vi "Get Visibility.vi"(8 "error in (no error)":errorcluster, 11 "Panel in":refnum<class "Panel.lvclass">) -> (0 "error out":errorcluster, 2 "Visible":bool, 3 "Panel out":refnum<class "Panel.lvclass">)   [LabVIEW 2018]
uses:
  Panel.lvclass
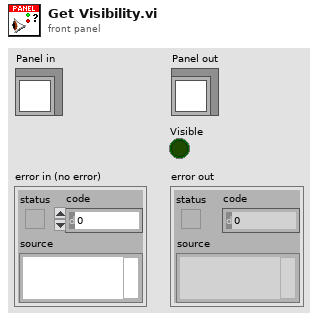
[diagram p1: front panel]
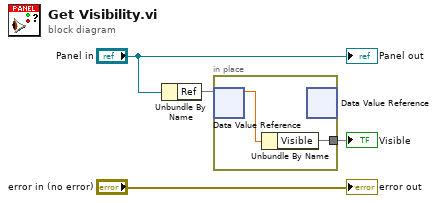
[diagram p0: block diagram]
diagram:
  n1 = Unbundle By Name("Panel in") -> ("Ref"=w3)
  n2 = in-place {
    in-place-border: [w5] -> w1
    n3 = in-place-dvr #1(w3) -> (w6:dbl)  [unwired: 1 out]
    n4 = Unbundle By Name(w6) -> ("Visible"=w5)
    n5 = in-place-dvr #1() -> ()  [unwired: 1 in, 2 out]
  }
  "Visible" <- w1
  "error out" <- "error in (no error)"
  "Panel out" <- "Panel in"
